vi "AS-Current-to-Pascals.vi"(10 "V0 In":dbl, 11 "V1 In":dbl) -> (2 "PA1 Out":dbl, 3 "PA0 Out":dbl)   [LabVIEW 2025]
uses:
  <vilib>/express/express arith-compare/Formula/XNode/ExpressFormulaBlockNode.xnode
panel:
  # "See block diagram for more information"
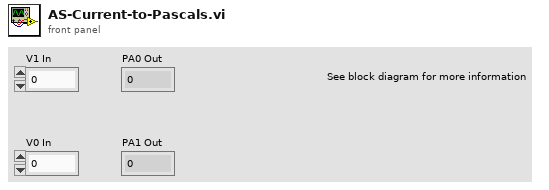
[diagram p1: front panel]
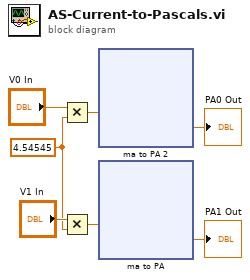
[diagram p0: block diagram]
diagram:
  w4 = 4.54545 ("y")
  n1 = Multiply(x="V0 In", y=w4) -> (x*y=w1:dbl)
  n2 = Multiply(x="V1 In", y=w4) -> (x*y=w2:dbl)
  n3 = xnode ("ma to PA 2")("ma"=w1) -> ("Result"=→"PA0 Out":dbl)  [unwired: 1 in, 1 out]
  n4 = xnode ("ma to PA")("ma"=w2) -> ("Result"=→"PA1 Out":dbl)  [unwired: 1 in, 1 out]
